vi "QCA Init Channels.vi"() -> ()   [LabVIEW 2019]
doc: "This VI reads the channel setup file and populates two arrays. First, an array containing all the fields (and their data types) that constitute a channel is filled. Second, an array containing values for each defined channel is filled from the contents of the setup file."
uses:
  e1039-target-controls/PDP/TPS Global.vi
  QCA Global.vi
  <vilib>/Utility/config.llb/NI_LVConfig.lvlib
panel:
  out "Array":string[][][](array[string])
  # "Channel #"
  # "Key #"
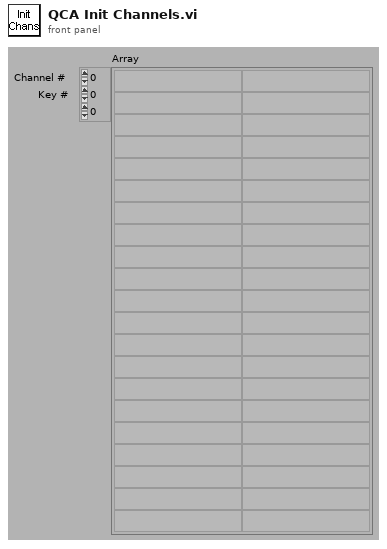
[diagram p1: front panel]
types:
  T1 = cluster{"Name":string, "Type":enum16{"I32", "DBL", "STR"}, "Changeable":bool}[]
  T2 = typedef "NI_LVConfig.lvlib/Config Data RefNum.ctl" = refnum<k1>
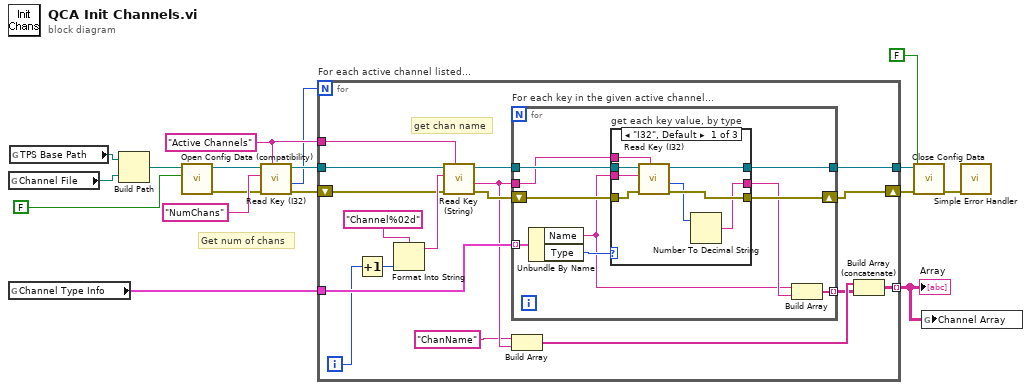
[diagram p0: block diagram]
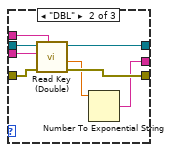
[diagram p2: hidden frame]
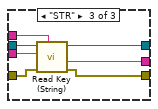
[diagram p3: hidden frame]
diagram:
  w12 = "Active Channels" ("section")
  # "Get num of chans"
  n1 = global read "QCA Global.vi" "Channel File"() -> (w2:path)
  n2 = global read "QCA Global.vi" "Channel Type Info"() -> (w3:T1)
  n3 = global read "TPS Global.vi" "TPS Base Path"() -> (w7:path)
  n4 = Build Path(base path=w7, name or relative path=w2) -> (appended path=w6:path)
  n5 = call <vilib>:"Open Config Data (compatibility).vi"("create file if necessary (T)"=FALSE ("create file if necessary? (T)"), "configuration file path"=w6) -> ("error out"=w14:errorcluster, "refnum"=w15:T2)  [unwired: 7 in, 1 out]
  n6 = call <vilib>:"Read Key (I32).vi"("section"=w12, "error in (no error)"=w14, "key"="NumChans", "refnum"=w15) -> ("error out"=w11:errorcluster, "value"=w4:i32, "refnum out"=w13:T2)  [unwired: 4 in, 1 out]
  n7 = for "For each active channel listed..." {
    N: w4 -> [_]
    tunnel: w13 -> [w32]
    tunnel: w12 -> [w31]
    shift-right: [w27] -> w10
    shift-left: w11 -> [w30]
    tunnel: w3 -> [w29]
    tunnel: [w25] -> w8
    tunnel: [w20] -> w5 mode=indexing
    i -> [w19]
    # "get chan name"
    n8 = Increment(x=w19) -> (x+1=w18:i32)
    n9 = Format Into String(format string="Channel%02d" ("Format String"), w18) -> (resulting string=w33:string)  [unwired: 2 in, 1 out]
    n10 = call <vilib>:"Read Key (String).vi"("section"=w31, "error in (no error)"=w30, "key"=w33, "refnum"=w32) -> ("error out"=w28:errorcluster, "value"=w24:string, "refnum out"=w26:T2)  [unwired: 4 in, 1 out]
    n11 = for "For each key in the given active channel..." {
      tunnel: w29 -> [w39] mode=indexing
      tunnel: w24 -> [w40]
      shift-right: [w42] -> w27
      shift-left: w28 -> [w43]
      tunnel: w26 -> [w44]
      tunnel: [w41] -> w25
      tunnel: [w35] -> w21 mode=indexing
      n12 = Unbundle By Name(w39) -> ("Name"=w36:string, "Type"=w38:enum16{"I32", "DBL", "STR"})
      n13 = case "get each key value, by type" shown="\"I32\", Default" w38 {
        tunnel: w44 -> [w52 w60 w67]
        tunnel: w43 -> [w51 w59 w66]
        tunnel: [w50 w58 w65] -> w42
        tunnel: [w49 w57 w64] -> w41
        tunnel: w40 -> [w48 w56 w63]
        tunnel: w36 -> [w47 w55 w62]
        tunnel: [w45 w53 w61] -> w37
        frame "I32", Default {
          n14 = call <vilib>:"Read Key (I32).vi"("section"=w48, "error in (no error)"=w51, "key"=w47, "refnum"=w52) -> ("error out"=w50:errorcluster, "value"=w46:i32, "refnum out"=w49:T2)  [unwired: 4 in, 1 out]
          n15 = Number To Decimal String(number=w46) -> (decimal integer string=w45:string)  [unwired: 1 in]
        }
        frame "DBL" {
          n16 = call <vilib>:"Read Key (Double).vi"("section"=w56, "error in (no error)"=w59, "key"=w55, "refnum"=w60) -> ("error out"=w58:errorcluster, "value"=w54:dbl, "refnum out"=w57:T2)  [unwired: 4 in, 1 out]
          n17 = Number To Exponential String(number=w54) -> (E-format string=w53:string)  [unwired: 3 in]
        }
        frame "STR" {
          n18 = call <vilib>:"Read Key (String).vi"("section"=w63, "error in (no error)"=w66, "key"=w62, "refnum"=w67) -> ("error out"=w65:errorcluster, "value"=w61:string, "refnum out"=w64:T2)  [unwired: 4 in, 1 out]
        }
      }
      n19 = Build Array(w36, w37) -> (w35:string[])
    }
    n20 = Build Array("ChanName" ("Input Element"), w24) -> (w22:string[])
    n21 = Build Array (concatenate)(w22, w21) -> (w20:string[][])
  }
  "Array" <- w5
  n22 = call <vilib>:"Close Config Data.vi"("error in (no error)"=w10, "write file if changed (T)"=FALSE, "refnum"=w8) -> ("error out"=w9:errorcluster)  [unwired: 7 in, 1 out]
  n23 = global write "QCA Global.vi" "Channel Array"(w5) -> ()
  n24 = call <vilib>:"Simple Error Handler.vi"("error in (no error)"=w9) -> ()  [unwired: 4 in, 5 out]
